vi "temperatureAlarmSystem.vi"() -> ()   [LabVIEW 2019]
panel:
  in  "open":bool
  in  "stop":bool
  out "light":bool
  in  "Slide":dbl(slide) scale=0.0..100.0
  out "Thermometer":dbl(slide) scale=0.0..100.0
  in  "String":string
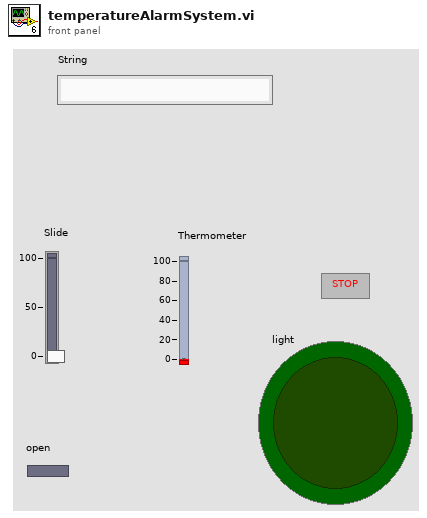
[diagram p1: front panel]
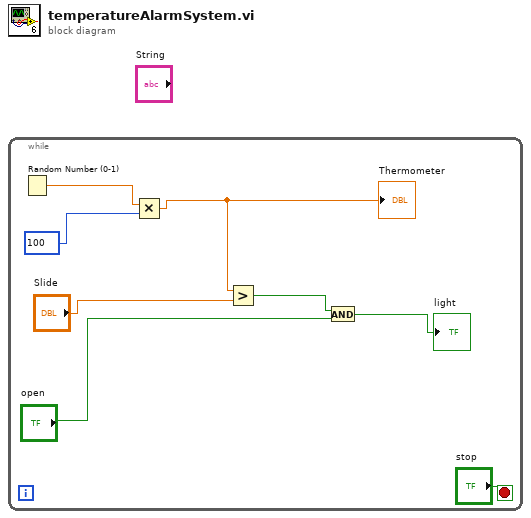
[diagram p0: block diagram]
diagram:
  n1 = while {
    stop <- "stop" stop-if-true
    n2 = Random Number (0-1)() -> (number: 0 to 1=w8:dbl)
    n3 = Multiply(x=w8, y=100) -> (x*y=w5:dbl)
    "Thermometer" <- w5
    n4 = Greater?(x=w5, y="Slide") -> (0:w4:bool)
    n5 = And(x=w4, y="open") -> (x .and. y?=→"light":bool)
  }
